vi "PyBoard <-> Spike BLE.vi"() -> ()   [LabVIEW 2016]
uses:
  VIs/uPythonX/uPythonX.xctl
panel:
  in  "Spike":T1(xcontrol)={"Port"="Spike - ASRL73::INSTR", "All Code"="import hub,utime\n\nhub.ble.scan(10)\n\nutime.sleep(10)\nhub.ble.scan_result()\n\n# wait a few seconds\np = hub.ble.connect(0) # hopefully index 0 is the pyboard, if not you'll have to find the right index via hub.ble.scan_result()\n\n# {'service_id': '232004FD-4200-0032-6670-6C2D64627970', 'rssi': -16, 'man_data': b'\\x00\\x00\\x80\\x98m\\x9a', 'mac_addr': '48:4A:30:01:9A:C2', 'man_id': 227}\n\n\np.callback(lambda data:print(data))\np.subscribe()\n\np.send('from hub')\n\np = hub.ble.connect(1)"}
  in  "PyBoard":T1(xcontrol)={"Port"="PyBoard - ASRL104::INSTR", "All Code"="import bluetooth\nbt = bluetooth.Bluetooth()\nbt.active(True)\n\nLPF2_SERVICE = bluetooth.UUID('00001623-1212-EFDE-1623-785FEABCD123')\nLWP_CHAR = (bluetooth.UUID('00001624-1212-EFDE-1623-785FEABCD123'), bluetooth.FLAG_NOTIFY|bluetooth.FLAG_WRITE,)\nlwp_char, = bt.gatts_add_service(LPF2_SERVICE, (LWP_CHAR,))\n\nbt.advertise(100, adv_data=bytearray('\\x02\\x01\\x02\\x0a\\x09pybd-lpf2'))\n\n\n\n#Now to send data from pyboard->hub do:\n\nbt.gatts_notify(lwp_char, 64, 'from pybd')\n\n#Then on pyboard get this data via:\n\nbt.gatts_read(lwp_char)\n\n# You can also register IRQ callbacks on the pyboard for all BLE events, like this:\n\n'''\ndef bt_irq(event, data):\n    print('bt_irq', event, data)\nbt.irq(bt_irq, bluetooth.IRQ_ALL)\n\n'''"}
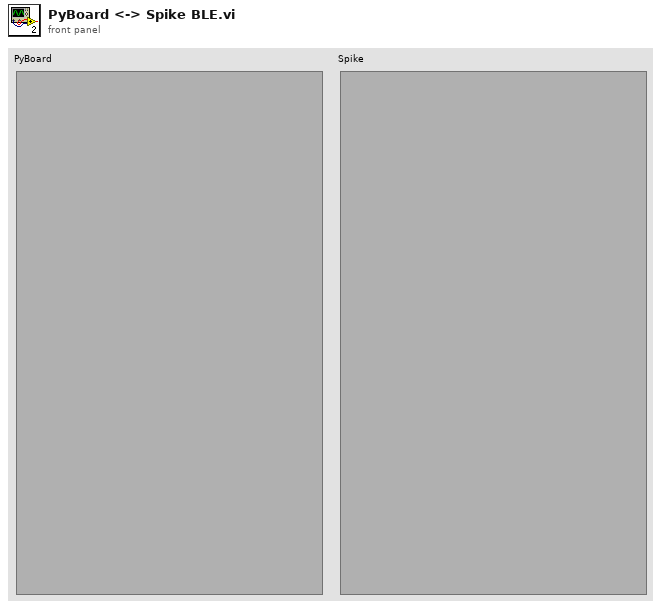
[diagram p1: front panel]
types:
  T1 = cluster{"Port":refnum<visa-resource-name>, "All Code":string}
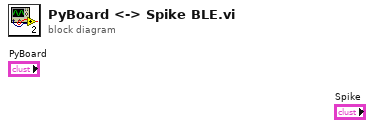
[diagram p0: block diagram]
diagram:
